vi "SaveMeasurementDataToFileSubVI.vi"(6 "Array of Time for Measurement":string[](array[string]), 7 "Array of Measurement":T1(array[cluster]), 8 "error in (no error)":errorcluster, 9 "Object number":string, 10 "Output Directory":path, 11 "VISA Refnum in":refnum<visa-resource-name>) -> (0 "error out":errorcluster, 3 "VISA Refnum out":refnum<visa-resource-name>)   [LabVIEW 2013]
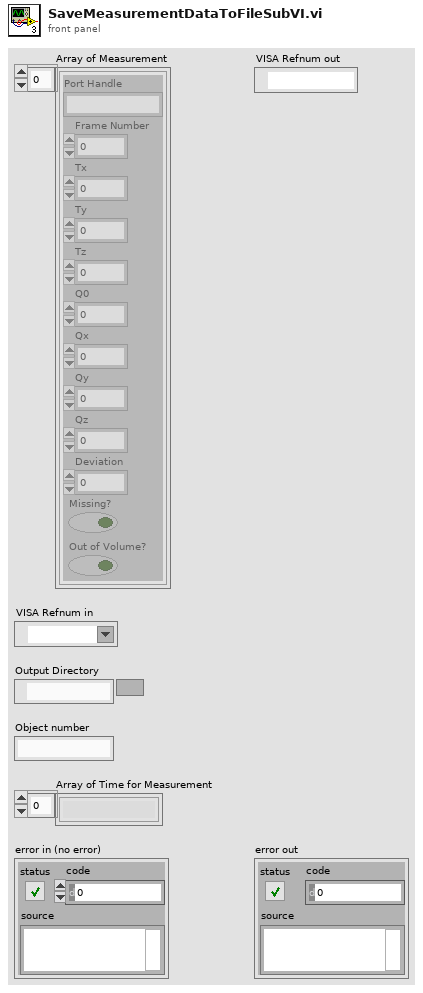
[diagram p1: front panel]
types:
  T1 = cluster{"Port Handle":string, "Frame Number":u32, "Tx":dbl, "Ty":dbl, "Tz":dbl, "Q0":dbl, "Qx":dbl, "Qy":dbl, "Qz":dbl, "Deviation":dbl, "Missing?":bool, "Out of Volume?":bool}[]
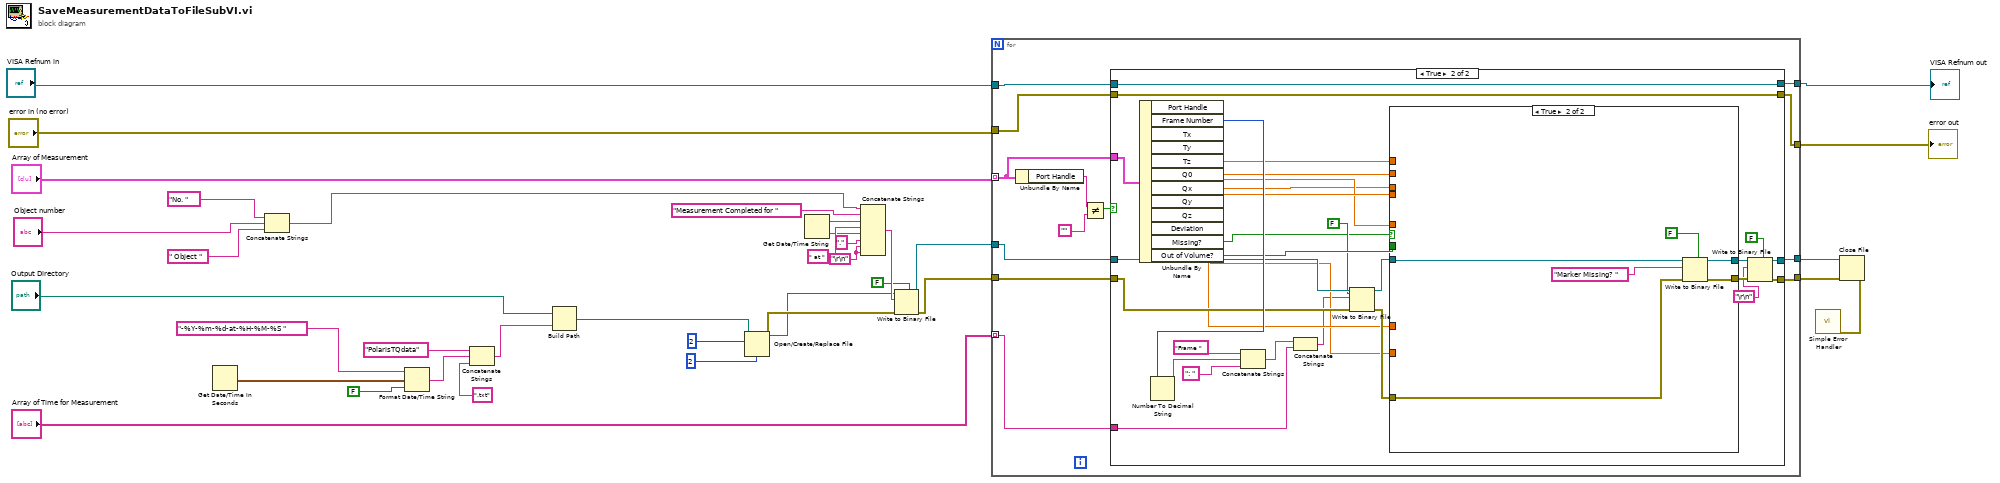
[diagram p0: block diagram]
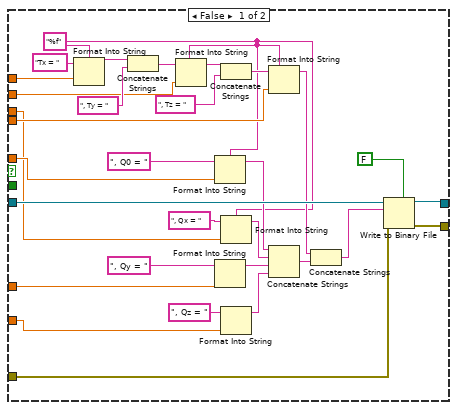
[diagram p3: hidden frame]
diagram:
  w27 = "\r\n"
  n1 = Get Date/Time In Seconds() -> (seconds since 1Jan1904=w19:timestamp)
  n2 = Concatenate Strings("No. ", "Object number", " Object ") -> (w5:string)
  n3 = Format Date/Time String(time format string (%c)="-%Y-%m-%d-at-%H-%M-%S ", seconds (now)=w19, UTC format=FALSE) -> (date/time string=w22:string)
  n4 = Concatenate Strings("PolarisTQdata", w22, ".txt") -> (w21:string)
  n5 = Build Path(base path="Output Directory", name or relative path=w21) -> (appended path=w20:path)
  n6 = Open/Create/Replace File(file path (use dialog)=w20, operation (0:open)=i8 2, access (0:read/write)=i8 2) -> (refnum out=w12:refnum<file>, error out=w13:errorcluster)  [unwired: 3 in, 1 out]
  n7 = Get Date/Time String() -> (date string=w32:string, time string=w30:string)  [unwired: 3 in]
  n8 = Concatenate Strings(w5, "Measurement Completed for ", w32, " at ", w30, "." ("string"), w27, w27) -> (w29:string)
  n9 = Write to Binary File(file (use dialog)=w12, data=w29, error in=w13, 5:FALSE ("prepend array or string size? (T)")) -> (refnum out=w10:refnum<file>, error out=w11:errorcluster)  [unwired: 2 in, 1 out]
  n10 = for {
    tunnel: w10 -> [w49]
    tunnel: [w47] -> w8
    tunnel: "Array of Measurement" -> [w41] mode=indexing
    tunnel: "Array of Time for Measurement" -> [w42] mode=indexing
    tunnel: "VISA Refnum in" -> [w40]
    tunnel: "error in (no error)" -> [w37]
    tunnel: [w39] -> w6
    tunnel: [w38] -> w1
    tunnel: w11 -> [w48]
    tunnel: [w46] -> w9
    n11 = Unbundle By Name(w41) -> ("Port Handle"=w45:string)
    n12 = Not Equal?(x=w45, y="") -> (x != y?=w44:bool)
    n13 = case shown="True" w44 {
      tunnel: w49 -> [w53 w82]
      tunnel: w48 -> [w52 w81]
      tunnel: [w53 w74] -> w47
      tunnel: [w52 w73] -> w46
      tunnel: w42 -> [_ w59]
      tunnel: w41 -> [_ w62]
      tunnel: w40 -> [w51 w56]
      tunnel: w37 -> [w50 w55]
      tunnel: [w51 w56] -> w39
      tunnel: [w50 w55] -> w38
      frame False {
      }
      frame True {
        n14 = Unbundle By Name(w62) -> ("Frame Number"=w83:u32, "Tx"=w78:dbl, "Ty"=w77:dbl, "Tz"=w76:dbl, "Q0"=w69:dbl, "Qx"=w68:dbl, "Qy"=w67:dbl, "Qz"=w66:dbl, "Missing?"=w54:bool, "Out of Volume?"=w72:bool)  [unwired: 2 out]
        n15 = Number To Decimal String(number=w83) -> (decimal integer string=w64:string)  [unwired: 1 in]
        n16 = Concatenate Strings("Frame ", w64, ": " ("string")) -> (w60:string)
        n17 = Concatenate Strings(w60, w59) -> (w61:string)
        n18 = Write to Binary File(file (use dialog)=w82, data=w61, error in=w81, 5:FALSE ("prepend array or string size? (T)")) -> (refnum out=w80:refnum<file>, error out=w79:errorcluster)  [unwired: 2 in, 1 out]
        n19 = case shown="True" w54 {
          tunnel: w80 -> [w103 w116]
          tunnel: w79 -> [w102 w117]
          tunnel: [w104 w120] -> w75
          tunnel: w78 -> [w113 _]
          tunnel: w77 -> [w109 _]
          tunnel: w76 -> [w105 _]
          tunnel: w72 -> [_ _]
          tunnel: w69 -> [w99 _]
          tunnel: w68 -> [w92 _]
          tunnel: w67 -> [w87 _]
          tunnel: w66 -> [w86 _]
          tunnel: [w84 w119] -> w57
          frame False {
            w94 = "%f" ("format string")
            n20 = Format Into String(format string=w94, initial string="Tx = ", w113) -> (resulting string=w112:string)  [unwired: 1 in, 1 out]
            n21 = Concatenate Strings(w112, ", Ty = ") -> (w110:string)
            n22 = Format Into String(format string=w94, initial string=w110, w109) -> (resulting string=w108:string)  [unwired: 1 in, 1 out]
            n23 = Format Into String(format string=w94, initial string=", Q0 = ", w99) -> (resulting string=w96:string)  [unwired: 1 in, 1 out]
            n24 = Format Into String(initial string=", Qy = ", w87) -> (resulting string=w91:string)  [unwired: 2 in, 1 out]
            n25 = Concatenate Strings(w108, ", Tz = ") -> (w107:string)
            n26 = Format Into String(format string=w94, initial string=", Qx = ", w92) -> (resulting string=w93:string)  [unwired: 1 in, 1 out]
            n27 = Format Into String(initial string=", Qz = ", w86) -> (resulting string=w90:string)  [unwired: 2 in, 1 out]
            n28 = Format Into String(format string=w94, initial string=w107, w105) -> (resulting string=w101:string)  [unwired: 1 in, 1 out]
            n29 = Concatenate Strings(w96, w93, w91, w90) -> (w97:string)
            n30 = Concatenate Strings(w101, w97) -> (w85:string)
            n31 = Write to Binary File(file (use dialog)=w103, data=w85, error in=w102, 5:FALSE ("prepend array or string size? (T)")) -> (refnum out=w84:refnum<file>, error out=w104:errorcluster)  [unwired: 2 in, 1 out]
          }
          frame True {
            n32 = Write to Binary File(file (use dialog)=w116, data="Marker Missing? ", error in=w117, 5:FALSE ("prepend array or string size? (T)")) -> (refnum out=w119:refnum<file>, error out=w120:errorcluster)  [unwired: 2 in, 1 out]
          }
        }
        n33 = Write to Binary File(file (use dialog)=w57, data="\r\n", error in=w75, 5:FALSE ("prepend array or string size? (T)")) -> (refnum out=w74:refnum<file>, error out=w73:errorcluster)  [unwired: 2 in, 1 out]
      }
    }
  }
  "VISA Refnum out" <- w6
  "error out" <- w1
  n34 = Close File(refnum=w8, error in=w9) -> (error out=w26:errorcluster)  [unwired: 1 out]
  n35 = call <vilib>:"Simple Error Handler.vi"("error in (no error)"=w26) -> ()  [unwired: 4 in, 5 out]
